vi "Execute Command.vi"   [LabVIEW 2015, in "SLSC Interface.lvclass"]
uses:
  SLSC Interface.lvclass
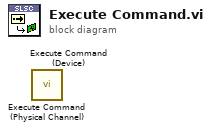
[diagram p0: block diagram]
diagram:
  n1 = call "Execute Command (Physical Channel).vi"() -> ()  [unwired: 14 in, 2 out]
  n2 = call "Execute Command (Device).vi"() -> ()  [unwired: 14 in, 2 out]
